vi "Power_errManu.vi"(3 "error in":errorcluster, 5 "addrPower":T1, 6 "pwr485":refnum<visa-resource-name>="COM3") -> (0 "error out":errorcluster, 1 "Message":string)   [LabVIEW 2015]
uses:
  CustomControl/addrPower.ctl
  <vilib>/Instr/_visa.llb/VISA Configure Serial Port (Instr).vi
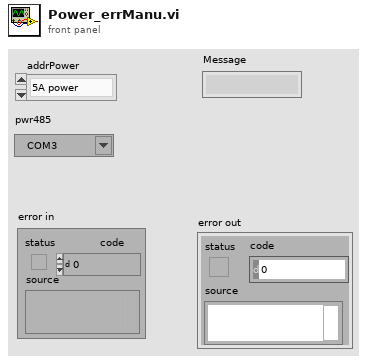
[diagram p1: front panel]
types:
  T1 = typedef "addrPower.ctl" = enum16{"5A power", "300A power"}
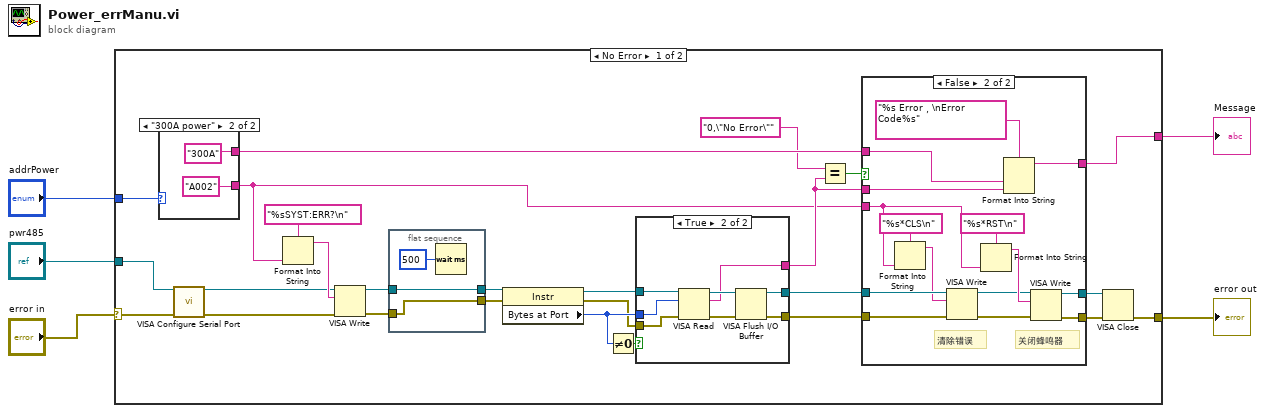
[diagram p0: block diagram]
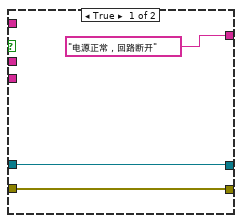
[diagram p2: hidden frame]
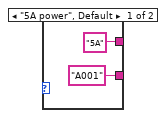
[diagram p4: hidden frame]
diagram:
  n1 = case shown="No Error" "error in" {
    selector: "error in" -> [w29 w67]
    tunnel: "pwr485" -> [w31 _]
    tunnel: [w30 w67] -> w4
    tunnel: "addrPower" -> [w7 _]
    tunnel: [w6 _] -> w1
    frame No Error {
      n2 = case shown="\"300A power\"" w7 {
        tunnel: ["A001" ("format string") "A002" ("format string")] -> w8
        tunnel: ["5A" ("format string") "300A" ("format string")] -> w22
        frame "5A power", Default {
        }
        frame "300A power" {
        }
      }
      n3 = call-poly "VISA Configure Serial Port"("VISA resource name"=w31, "error in (no error)"=w29) -> ("VISA resource name out"=w17:refnum<visa-resource-name>, "error out"=w16:errorcluster)  [unwired: 12 in]
      n4 = Format Into String(format string="%sSYST:ERR?\n", w8) -> (resulting string=w27:string)  [unwired: 2 in, 1 out]
      n5 = VISA Write(VISA resource name=w17, write buffer=w27, error in (no error)=w16) -> (VISA resource name out=w15:refnum<visa-resource-name>, error out=w14:errorcluster)  [unwired: 1 out]
      n6 = flat-sequence {
        tunnel: w15 -> [w33]
        tunnel: w14 -> [w32]
        tunnel: [w33] -> w13
        tunnel: [w32] -> w12
        frame #0 {
          n7 = Wait (ms)(milliseconds to wait=u32 500) -> ()  [unwired: 1 out]
        }
      }
      n8 = property class="Instr"(reference=w13, error in=w12) -> (reference out=w24:refnum<visa-resource-name>, error out=w23:errorcluster, "Bytes at Port"=w25:u32)
      n9 = Not Equal To 0?(x=w25) -> (x != 0?=w26:bool)
      n10 = case shown="True" w26 {
        tunnel: w25 -> [_ w62]
        tunnel: w24 -> [w54 w61]
        tunnel: w23 -> [w53 w60]
        tunnel: [w54 w57] -> w21
        tunnel: [w53 w56] -> w20
        tunnel: [_ w55] -> w9
        frame False {
        }
        frame True {
          n11 = VISA Read(VISA resource name=w61, byte count=w62, error in (no error)=w60) -> (VISA resource name out=w58:refnum<visa-resource-name>, read buffer=w55:string, error out=w59:errorcluster)  [unwired: 1 out]
          n12 = VISA Flush I/O Buffer(VISA resource name=w58, error in (no error)=w59) -> (VISA resource name out=w57:refnum<visa-resource-name>, error out=w56:errorcluster)  [unwired: 1 in]
        }
      }
      n13 = Equal?(x="0,\"No Error\"", y=w9) -> (x = y?=w11:bool)
      n14 = case shown="False" w11 {
        tunnel: w22 -> [_ w47]
        tunnel: w21 -> [w37 w50]
        tunnel: w20 -> [w36 w49]
        tunnel: [w37 w42] -> w19
        tunnel: [w36 w41] -> w18
        tunnel: w9 -> [_ w40]
        tunnel: w8 -> [_ w39]
        tunnel: ["电源正常，回路断开" ("message") w38] -> w6
        frame True {
        }
        frame False {
          # "关闭蜂鸣器"
          # "清除错误"
          n15 = Format Into String(format string="%s*CLS\n", w39) -> (resulting string=w48:string)  [unwired: 2 in, 1 out]
          n16 = VISA Write(VISA resource name=w50, write buffer=w48, error in (no error)=w49) -> (VISA resource name out=w44:refnum<visa-resource-name>, error out=w43:errorcluster)  [unwired: 1 out]
          n17 = Format Into String(format string="%s*RST\n", w39) -> (resulting string=w45:string)  [unwired: 2 in, 1 out]
          n18 = Format Into String(format string="%s Error，\nError Code%s", w47, w40) -> (resulting string=w38:string)  [unwired: 2 in, 1 out]
          n19 = VISA Write(VISA resource name=w44, write buffer=w45, error in (no error)=w43) -> (VISA resource name out=w42:refnum<visa-resource-name>, error out=w41:errorcluster)  [unwired: 1 out]
        }
      }
      n20 = VISA Close(VISA resource name=w19, error in (no error)=w18) -> (error out=w30:errorcluster)
    }
    frame Error {
    }
  }
  "error out" <- w4
  "Message" <- w1
